vi "LogMessage.vi"(8 "error in (no error)":errorcluster, 9 "Verbosity":T1=enum."Default", 10 "Message":string, 11 "Logger in":refnum<class "Logger.lvclass">) -> (0 "error out":errorcluster, 3 "Logger out":refnum<class "Logger.lvclass">)   [LabVIEW 2014, in "Logger.lvclass"]
uses:
  Logger.lvclass
  Verbosity.ctl
  Logger.lvclass/Logger.ctl
  <vilib>/ErrorRing/Error Ring.xnode
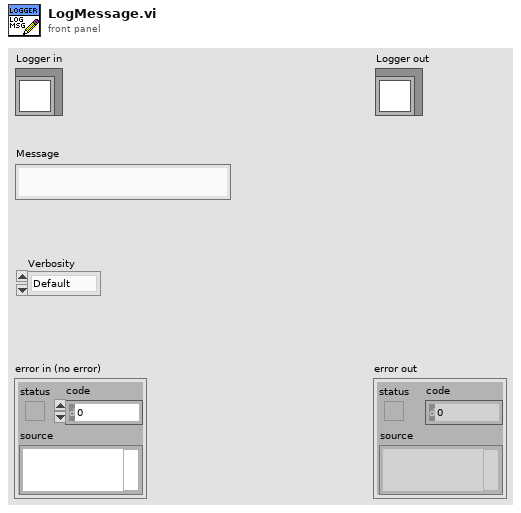
[diagram p1: front panel]
types:
  T1 = typedef "Verbosity.ctl" = enum16{"Minimal", "Default", "Detailed", "Diagnostic"}
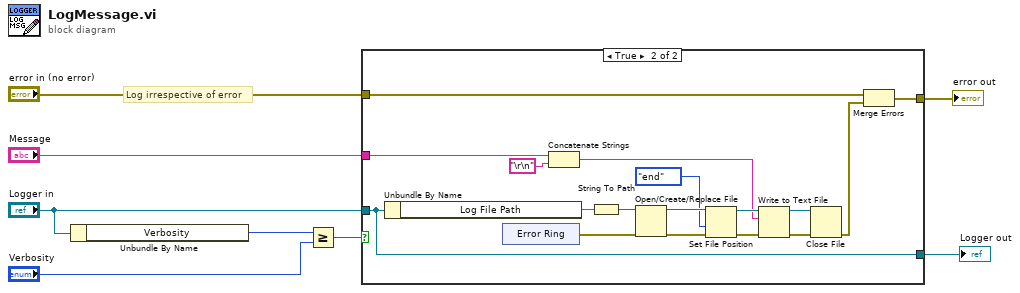
[diagram p0: block diagram]
diagram:
  # "Log irrespective of error"
  n1 = Unbundle By Name("Logger in") -> ("Verbosity"=w1:T1)
  n2 = Greater Or Equal?(x=w1, y="Verbosity") -> (x >= y?=w3:bool)
  n3 = case shown="True" w3 {
    tunnel: [w9 w27] -> w8
    tunnel: "Logger in" -> [w10 w14]
    tunnel: "error in (no error)" -> [w9 w13]
    tunnel: "Message" -> [_ w26]
    tunnel: [w10 w14] -> w5
    frame False {
    }
    frame True {
      n4 = Unbundle By Name(w14) -> ("Log File Path"=w25:string)
      n5 = xnode "Error Ring"() -> ("error out"=w15:errorcluster)
      n6 = Concatenate Strings(w26, "\r\n") -> (w17:string)
      n7 = String To Path(string=w25) -> (path=w11:path)
      n8 = Open/Create/Replace File(file path (use dialog)=w11, error in=w15) -> (refnum out=w20:refnum<file>, error out=w24:errorcluster)  [unwired: 4 in, 1 out]
      n9 = Set File Position(refnum=w20, from (0:start)=enum16{"start", "end", "current"}."end", error in=w24) -> (refnum out=w19:refnum<file>, error out=w21:errorcluster)  [unwired: 1 in]
      n10 = Write to Text File(file (use dialog)=w19, text=w17, error in=w21) -> (refnum out=w22:refnum<file>, error out=w23:errorcluster)  [unwired: 1 in, 1 out]
      n11 = Close File(refnum=w22, error in=w23) -> (error out=w12:errorcluster)  [unwired: 1 out]
      n12 = Merge Errors(w13, w12) -> (w27:errorcluster)
    }
  }
  "error out" <- w8
  "Logger out" <- w5
